vi "AB_Set_Password_CORE.vi"(8 "error in (no error)":errorcluster, 9 "Password setting":T1, 10 "Password":string, 11 "Source in":refnum<class "AB_Source.lvclass">) -> (0 "error out":errorcluster, 3 "Source out":refnum<class "AB_Source.lvclass">)   [LabVIEW 2020]
uses:
  <vilib>/AppBuilder/AB_Password_Setting.ctl
  <vilib>/AppBuilder/AB_Classes/Source/AB_Source.lvclass
  <vilib>/AppBuilder/AB_Source_Property_Type.ctl
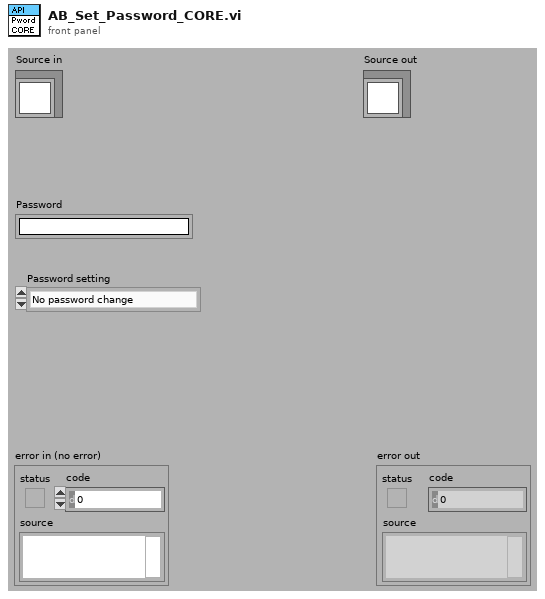
[diagram p1: front panel]
types:
  T1 = typedef "AB_Password_Setting.ctl" = enum32{"No password change", "Remove password", "Apply new password"}
  T2 = typedef "AB_Source_Property_Type.ctl" = enum16{"Remove block diagram", "Remove front panel", "Password", "Window has title bar", "Show menu bar", "Show vertical scroll bar", "Show horizontal scroll bar", "Show toolbar", "Show Abort button", "Show fp when called", "Window behavior", "Allow user to close window", "Window run-time position", "Run when opened", "Allow debugging", "Auto error handling", "Generate guard code", "Use stack variables", "Expression folding", "Integer only", "Inline subVI"}
  T3 = typedef "AB_Source.ctl" = cluster{"path":path, "itemID":string, "parentIndex":i32, "sourceInclusion":T4, "destinationIndex":i32, "properties":T5[], "newName":string, "lvfile":bool, "valid":bool, "eng_inBuild":bool, "eng_isNonVILink":bool, "Amalgamation":bool, "Amalgamation Piece":bool, "eng_delimitedName":string, "preventRename":bool}
  T4 = typedef "AB_Source_Inclusion.ctl" = enum16{"IncludeIfReferenced", "Include", "Exclude", "TopLevel"}
  T5 = typedef "AB_Source_Properties.ctl" = cluster{"sourcePropertyType":T2, "value":variant}
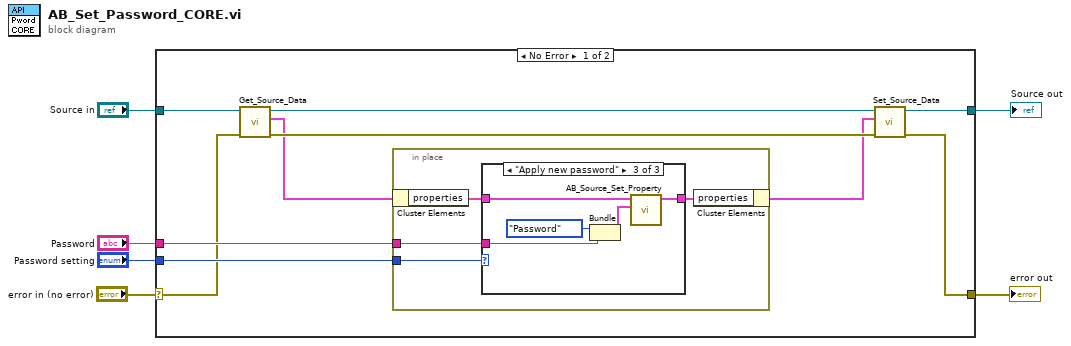
[diagram p0: block diagram]
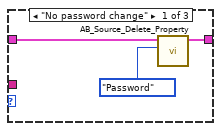
[diagram p2: hidden frame]
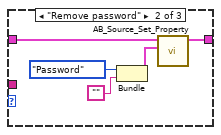
[diagram p3: hidden frame]
diagram:
  n1 = case shown="No Error" "error in (no error)" {
    selector: "error in (no error)" -> [w8 w35]
    tunnel: [w7 w35] -> w5
    tunnel: "Password" -> [w12 _]
    tunnel: "Password setting" -> [w11 _]
    tunnel: [w10 w34] -> w2
    tunnel: "Source in" -> [w9 w34]
    frame No Error {
      n2 = call <vilib>:"Get_Source_Data.vi"("error in (no error)"=w8, "Class in"=w9) -> ("error out"=w15:errorcluster, "data"=w14:T3, "Class out"=w16:refnum<class "AB_Source.lvclass">)  [unwired: 7 out]
      n3 = in-place {
        in-place-border: w11 -> [w20]
        in-place-border: w12 -> [w17]
        n4 = in-place-cluster #1(w14) -> ("properties"=w19:T5[])
        n5 = case shown="\"Apply new password\"" w20 {
          tunnel: w19 -> [w22 w26 w32]
          tunnel: [w21 w24 w30] -> w18
          tunnel: w17 -> [_ _ w29]
          frame "No password change" {
            n6 = call <vilib>:"AB_Source_Delete_Property.vi"("type"=AB_Source_Property_Type."Password", "sourceProperties in"=w22) -> ("sourceProperties out"=w21:T5[])  [unwired: 1 in, 8 out]
          }
          frame "Remove password" {
            n7 = Bundle("y"=AB_Source_Property_Type."Password", "") -> (w25:cluster{"y":T2, string})  [unwired: 1 out]
            n8 = call <vilib>:"AB_Source_Set_Property.vi"("sourceProperty"=w25, "sourceProperties in"=w26) -> ("sourceProperties out"=w24:T5[])  [unwired: 1 in, 8 out]
          }
          frame "Apply new password" {
            n9 = Bundle("y"=AB_Source_Property_Type."Password", "Password"=w29) -> (w31:cluster{"y":T2, "Password":string})  [unwired: 1 out]
            n10 = call <vilib>:"AB_Source_Set_Property.vi"("sourceProperty"=w31, "sourceProperties in"=w32) -> ("sourceProperties out"=w30:T5[])  [unwired: 1 in, 8 out]
          }
        }
        n11 = in-place-cluster #1("properties"=w18) -> (w13:T3)
      }
      n12 = call <vilib>:"Set_Source_Data.vi"("error in (no error)"=w15, "data"=w13, "Class in"=w16) -> ("error out"=w7:errorcluster, "Class out"=w10:refnum<class "AB_Source.lvclass">)  [unwired: 7 out]
    }
    frame Error {
    }
  }
  "error out" <- w5
  "Source out" <- w2
